vi "ParseResponseSDIO.vi"(8 "error in (no error)":errorcluster, 11 "Value":string) -> (0 "error out":errorcluster, 2 "status":string, 3 "description":string)   [LabVIEW 2021]
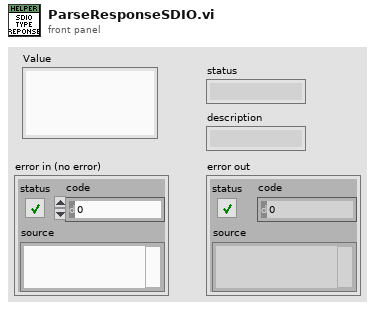
[diagram p1: front panel]
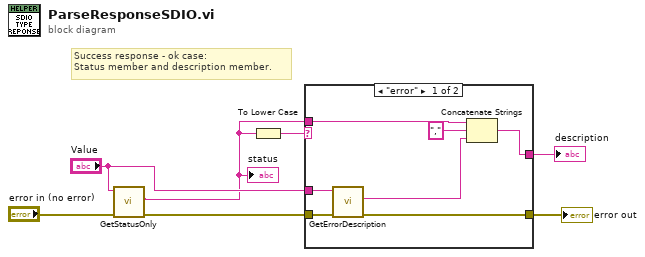
[diagram p0: block diagram]
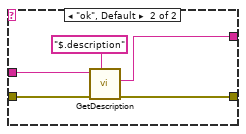
[diagram p2: hidden frame]
diagram:
  # "Success response - ok case:\nStatus member and description member."
  n1 = call "GetStatusOnly.vi"("error in (no error)"="error in (no error)", "Value"="Value") -> ("error out"=w5:errorcluster, "status"=w1:string)  [unwired: 7 in, 1 out]
  "status" <- w1
  n2 = To Lower Case(string=w1) -> (all lower case string=w2:string)
  n3 = case shown="\"error\"" w2 {
    tunnel: [w12 w16] -> w4
    tunnel: "Value" -> [w14 w18]
    tunnel: w5 -> [w13 w19]
    tunnel: [w9 w17] -> w3
    tunnel: w1 -> [w8 _]
    frame "error" {
      n4 = call "GetErrorDescription.vi"("error in (no error)"=w13, "Value"=w14) -> ("error out"=w12:errorcluster, "description"=w10:string)  [unwired: 7 in, 1 out]
      n5 = Concatenate Strings(w8, "," ("string"), w10) -> (w9:string)
    }
    frame "ok", Default {
      n6 = call "GetDescription.vi"("$Path or Item Name"="$.description", "error in (no error)"=w19, "Value"=w18) -> ("error out"=w16:errorcluster, "description"=w17:string)  [unwired: 7 in]
    }
  }
  "error out" <- w4
  "description" <- w3
